vi "SQL_test_Template_selectbyname.vi"(11 "模板名称":string) -> (0 "error out":errorcluster, 3 "载荷谱信息":string[][](table))   [LabVIEW 2014]
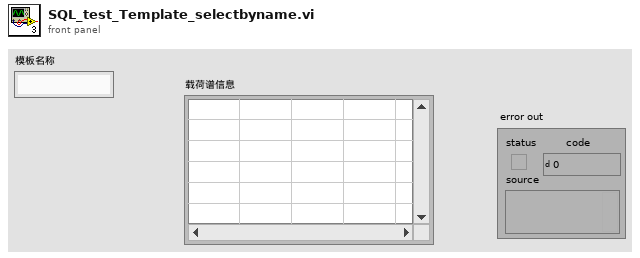
[diagram p1: front panel]
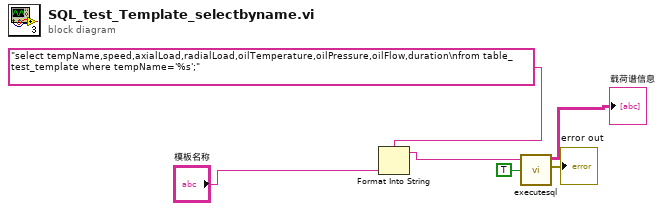
[diagram p0: block diagram]
diagram:
  n1 = Format Into String(format string="select tempName,speed,axialLoad,radialLoad,oilTemperature,oilPressure,oilFlow,duration\nfrom table_test_template where tempName='%s';", "模板名称") -> (resulting string=w4:string)  [unwired: 2 in, 1 out]
  n2 = call "executesql.vi"("Return Data (T)"=TRUE, "Command Text"=w4) -> ("error out"=→"error out":errorcluster, "Data"=→"载荷谱信息":string[][])  [unwired: 5 in]
